vi "Curvature of Bezier Spline.vi"(11 "bezier spline waypts":T1) -> (3 "curvature":dbl[][](array[numeric]))   [LabVIEW 2019]
uses:
  Types/Bezier Spline.ctl
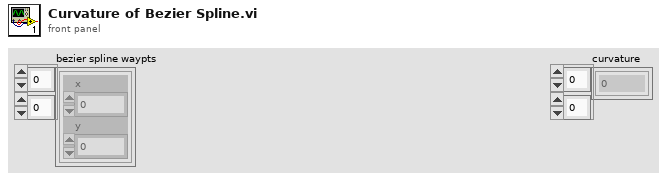
[diagram p1: front panel]
types:
  T1 = typedef "Bezier Spline.ctl" = cluster{"x":dbl, "y":dbl}[][]
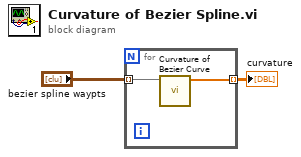
[diagram p0: block diagram]
diagram:
  n1 = for {
    tunnel: "bezier spline waypts" -> [w4] mode=indexing
    tunnel: [w3] -> w1 mode=indexing
    n2 = call "Curvature of Bezier Curve.vi"("curve"=w4) -> ("curvature"=w3:dbl[])  [unwired: 10 in]
  }
  "curvature" <- w1
